vi "add vi reference to all CSM Modules.vi"() -> ()   [LabVIEW 2017]
uses:
  user.lib/_NEVSTOP/Communicable State Machine(CSM)/_csmHelper/CSM-Helper.lvclass/CSM-Helper.ctl
  user.lib/_NEVSTOP/Communicable State Machine(CSM)/_csmHelper/Properties/Read Parse State Queue Ref.vi
  user.lib/_NEVSTOP/Communicable State Machine(CSM)/_csmHelper/API/Destroy.vi
  user.lib/_NEVSTOP/Communicable State Machine(CSM)/_csmHelper/CSM-Helper.lvclass
panel:
  out "Array":cluster{path, "error out":errorcluster}[](array[cluster])
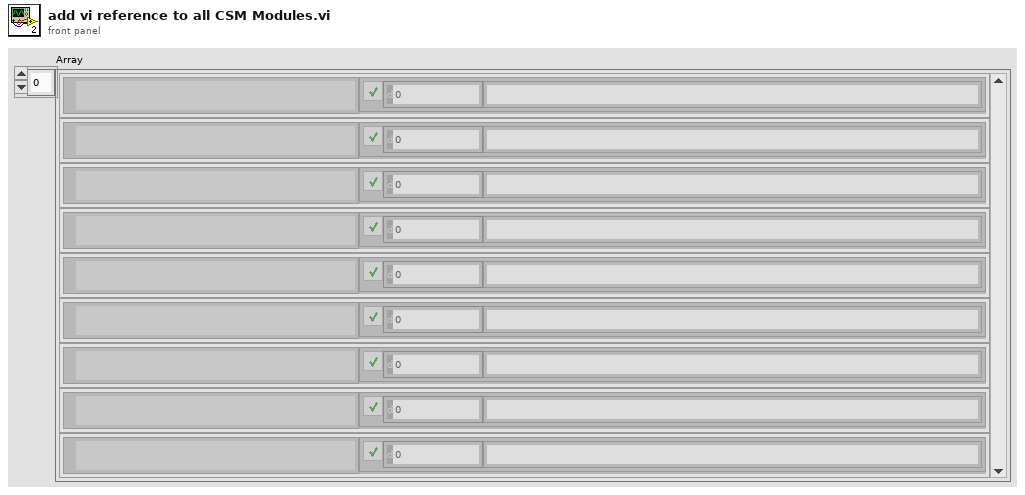
[diagram p1: front panel]
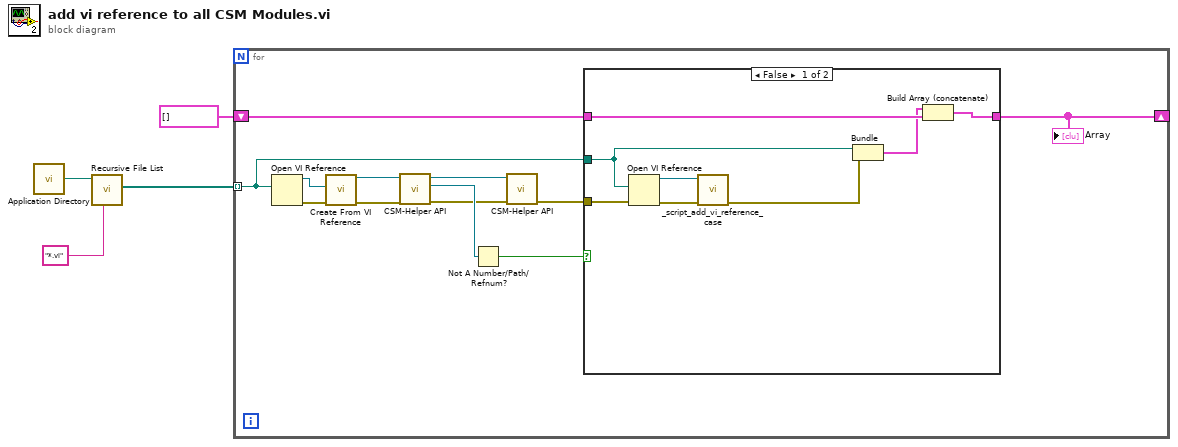
[diagram p0: block diagram]
diagram:
  n1 = call <vilib>:"Application Directory.vi"() -> ("Application Directory"=w4:path)
  n2 = call <vilib>:"Recursive File List.vi"("pattern"="*.vi", "Folder Path"=w4) -> ("All Files in Dir"=w2:path[])  [unwired: 5 in, 4 out]
  n3 = for {
    tunnel: w2 -> [w7] mode=indexing
    shift-right: [w6] -> _
    shift-left: cluster{path, "error out":errorcluster}[] [] -> [w5]
    n4 = Open VI Reference(vi path=w7) -> (vi reference=w15:refnum<vi>, error out=w16:errorcluster)  [unwired: 5 in]
    n5 = call "Create From VI Reference.vi"("error in (no error)"=w16, "VI"=w15) -> ("error out"=w14:errorcluster, "CSM-Helper.lvclass"=w13:refnum<class "CSM-Helper.lvclass">)  [unwired: 8 in]
    n6 = call-poly "CSM-Helper API.vi"("error in (no error)"=w14, "CSM-Helper in"=w13) -> ("error out"=w11:errorcluster, "Parse State Queue"=w12:refnum<vi>, "CSM-Helper out"=w10:refnum<class "CSM-Helper.lvclass">)  [unwired: 7 in]
    n7 = Not A Number/Path/Refnum?(number/path/refnum=w12) -> (NaN/Path/Refnum?=w8:bool)
    n8 = call-poly "CSM-Helper API.vi"("error in (no error)"=w11, "CSM-Helper in"=w10) -> ("error out"=w9:errorcluster)  [unwired: 8 in, 1 out]
    n9 = case shown="False" w8 {
      tunnel: w9 -> [w24 _]
      tunnel: w7 -> [w21 _]
      tunnel: [w19 w25] -> w6
      tunnel: w5 -> [w18 w25]
      frame False {
        n10 = Open VI Reference(vi path=w21, error in (no error)=w24) -> (vi reference=w23:refnum<vi>, error out=w22:errorcluster)  [unwired: 4 in]
        n11 = call "_script_add_vi_reference_case.vi"("error in (no error)"=w22, "reference"=w23) -> ("error out"=w20:errorcluster)  [unwired: 9 in]
        n12 = Bundle(w21, "error out"=w20) -> (w17:cluster{path, "error out":errorcluster})  [unwired: 1 in]
        n13 = Build Array (concatenate)(w17, w18) -> (w19:cluster{path, "error out":errorcluster}[])
      }
      frame True {
      }
    }
    "Array" <- w6
  }
